vi "AVS_GetLambda.vi"(0 "a_hDevice":i32, 11 "a_pWaveLength":dbl[](array[numeric])) -> (4 "Output Value":i32, 15 "a_pWaveLength":dbl[](array[numeric]))   [LabVIEW 2013, in "Avantes Spectrometer Functions.lvlib"]
uses:
  Avantes Spectrometer Functions.lvlib
  AvantesSpectrometer2/polling_mc/AS5216.dll
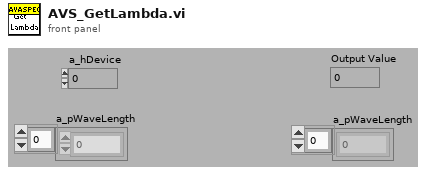
[diagram p1: front panel]
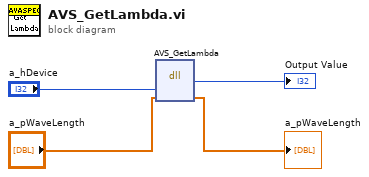
[diagram p0: block diagram]
diagram:
  n1 = dll-call lib="C:/Users/dhstuart/Dropbox/CLTC/AvantesSpectrometer2/polling_mc/AS5216.dll" fn="AVS_GetLambda"("a_hDevice"="a_hDevice", "a_pWaveLength"="a_pWaveLength") -> (→"Output Value":i32, "a_pWaveLength"=→"a_pWaveLength":dbl[])  [unwired: 4 in, 2 out]
